vi "blood pressure MAP detection fromdata.vi"() -> ()   [LabVIEW 2019]
uses:
  <vilib>/Analysis/3filter.llb/Filter Passband Type.ctl
  <vilib>/Analysis/3filter.llb/Butterworth Filter (DBL).vi
  <vilib>/Analysis/NI_AALBase.lvlib
panel:
  out "Waveform Graph":dbl[](graph)
  out "Index of Max":dbl
  out "Maximum after Gate":dbl
  out "MAP":dbl[](array[numeric])
  out "XY Graph":cluster{"Array":dbl[], "Filtered X":dbl[]}(graph)
  out "Filtered sig":dynamicdata(graph)
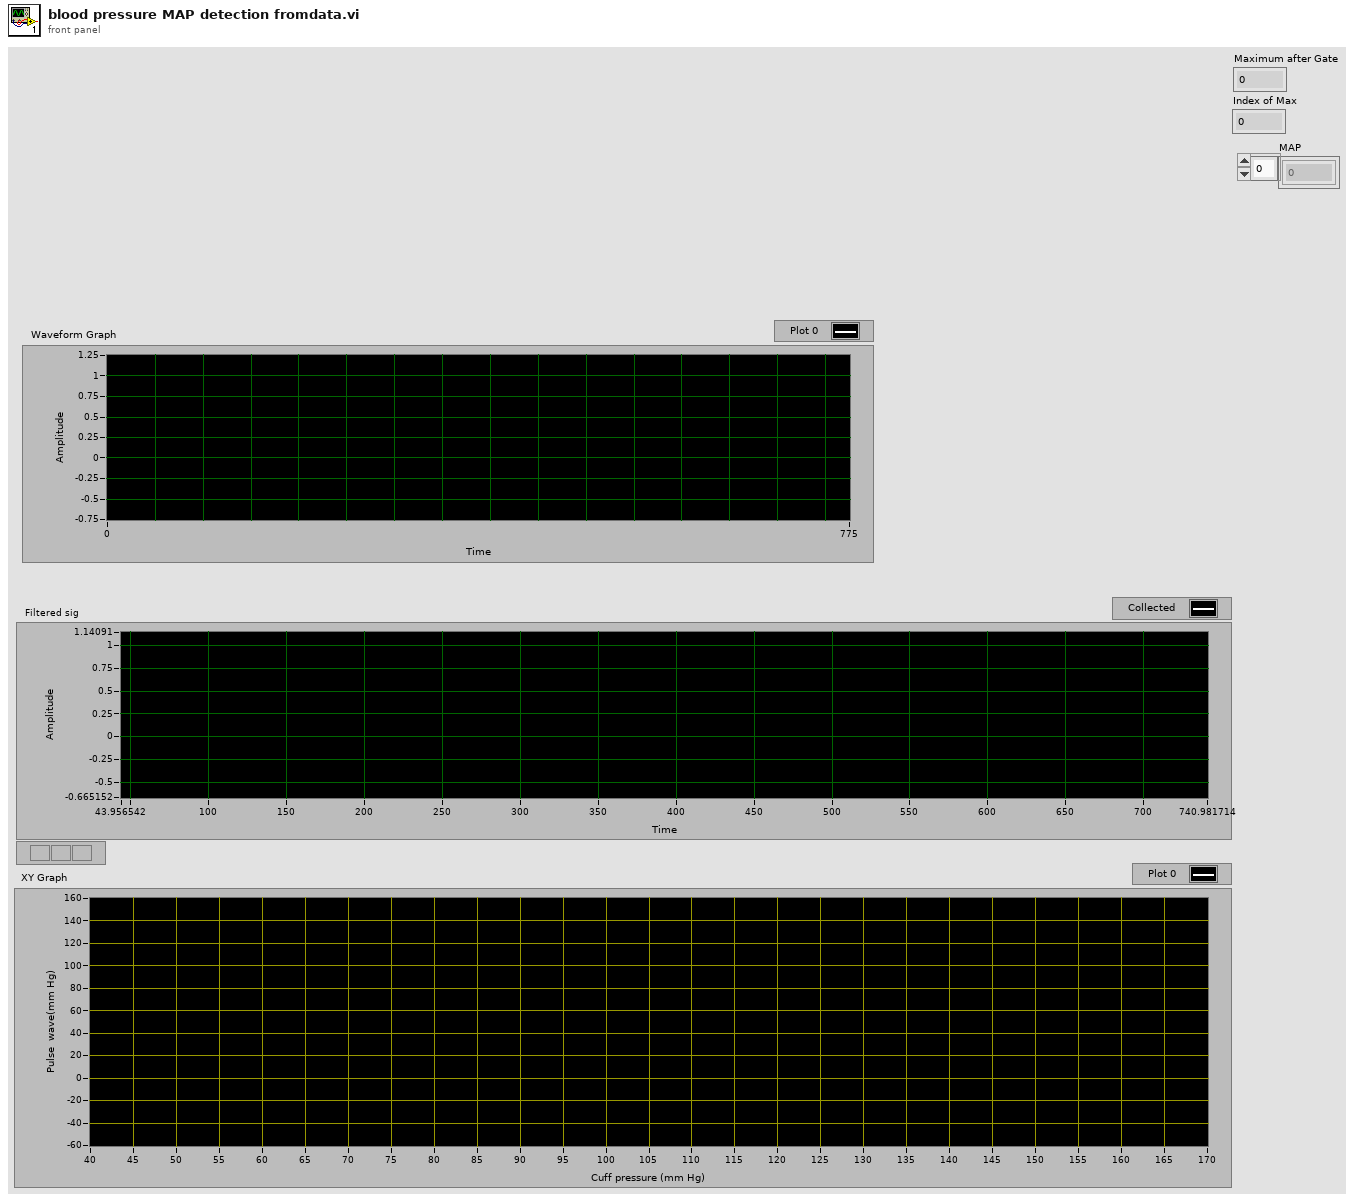
[diagram p1: front panel]
types:
  T1 = typedef "NI_AALBase.lvlib/Filter Passband Type.ctl" = enum32{"Lowpass", "Highpass", "Bandpass", "Bandstop"}
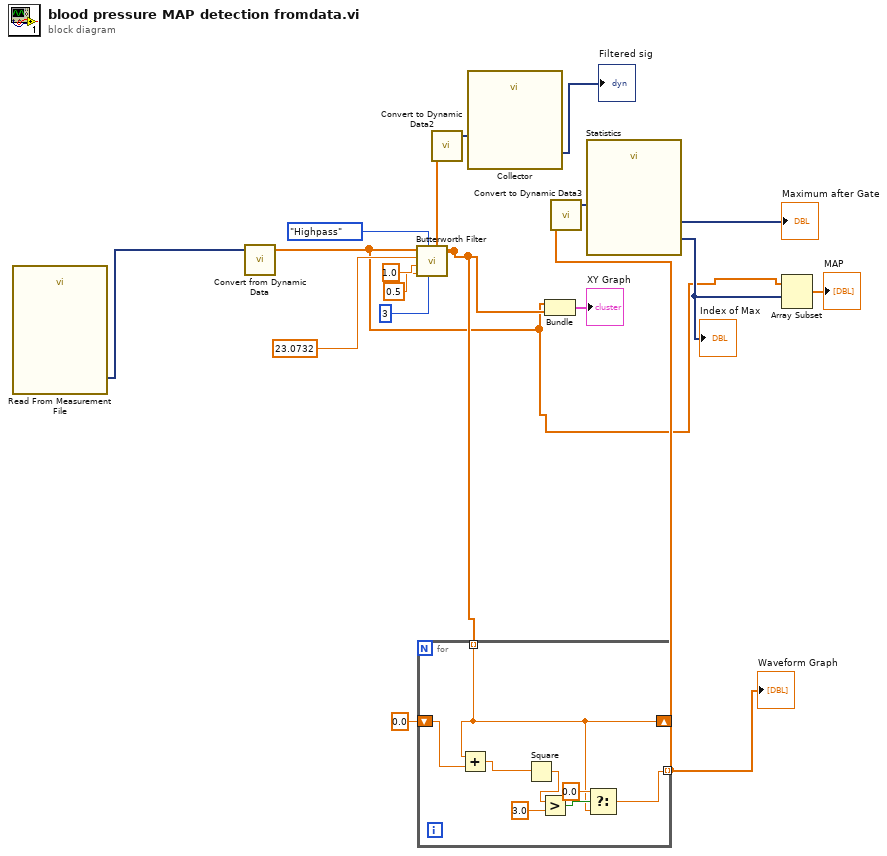
[diagram p0: block diagram]
diagram:
  n1 = call "Read From Measurement File"() -> ("Signals"=w10:dynamicdata)  [unwired: 6 in, 5 out]
  n2 = call "Convert from Dynamic Data"("Dynamic Data Type"=w10) -> ("Array"=w1:dbl[])  [unwired: 3 in]
  n3 = call-poly <vilib>:"Butterworth Filter.vi"("order"=3, "filter type"=Filter_Passband_Type."Highpass", "low cutoff freq: fl"=0.5, "high cutoff freq: fh"=1.0, "sampling freq: fs"=23.0732, "X"=w1) -> ("Filtered X"=w4:dbl[])  [unwired: 2 in, 1 out]
  n4 = for {
    tunnel: w4 -> [w19] mode=indexing
    shift-right: [w19] -> _
    shift-left: 0.0 -> [w25]
    tunnel: [w18] -> w3 mode=indexing
    n5 = Add(x=w19, y=w25) -> (x+y=w24:dbl)
    n6 = Square(x=w24) -> (x^2=w23:dbl)
    n7 = Greater?(x=w23, y=3.0) -> (0:w21:bool)
    n8 = Select(t=0.0, s=w21, f=w19) -> (s? t:f=w18:dbl)
  }
  "Waveform Graph" <- w3
  n9 = call "Convert to Dynamic Data2"("Array"=w4) -> ("Dynamic Data Type"=w8:dynamicdata)  [unwired: 3 in]
  n10 = call "Collector"("Signals"=w8) -> ("Collected Signals"=→"Filtered sig":dynamicdata)  [unwired: 9 in, 1 out]
  n11 = Bundle("Array"=w1, "Filtered X"=w4) -> (→"XY Graph":cluster{"Array":dbl[], "Filtered X":dbl[]})  [unwired: 1 in]
  n12 = call "Convert to Dynamic Data3"("Array"=w3) -> ("Dynamic Data Type"=w2:dynamicdata)  [unwired: 3 in]
  n13 = call "Statistics"("Signals"=w2) -> ("Index of Max"=w13:dynamicdata, "Maximum"=→"Maximum after Gate":dynamicdata)  [unwired: 24 in, 1 out]
  "Index of Max" <- w13
  n14 = Array Subset(array=w1, index=w13) -> (→"MAP":dbl[])  [unwired: 1 in]
